vi "FPGAmain_5782_Dual_PID_3.vi"() -> ()   [LabVIEW 2013]
uses:
  FPGA/DataMode.ctl
  FPGA/Input_5782/5782_states.ctl
  <vilib>/Platform/TimedLoop/XDataNode/timing_clust.ctl
  <vilib>/Platform/TimedLoop/XDataNode/nitl_modes.ctl
  <vilib>/Platform/TimedLoop/XDataNode/wakeup.ctl
  <vilib>/rvi/Emulation/niFpgaSctlEmulationGetInTimedLoop.vi
  <vilib>/rvi/Emulation/niFpgaEmulationReportErrorSimple.vi
  <vilib>/rvi/Emulation/niFpgaGetClockAttributes.vi
  <vilib>/rvi/eio/common/nirviEmuTemplateMethod_errors.vi
  <vilib>/rvi/Emulation/niFpgaCriticalErrorInLSC.vi
  <vilib>/rvi/DataTransferAndStorage/Register/Emulation/niFpgaRegisterEmulationFpgaImpl.vi
  <instcachedir>/0/niFpgaRegisterEmulationFpgaImpl_DCF4BC0110594B98B44A971D60CEEC4D.lvgen/niFpgaRegisterEmulationFpgaImpl_DCF4BC0110594B98B44A971D60CEEC4D_005.vi
  <vilib>/rvi/DataTransferAndStorage/Container/Common/niFpgaContainerGetUniqueNameForEmu.vi
  <instcachedir>/0/niFpgaRegisterEmulationFpgaImpl_DCF4BC0110594B98B44A971D60CEEC4D.lvgen/niFpgaRegisterEmulationFpgaImpl_DCF4BC0110594B98B44A971D60CEEC4D_014.vi
  <instcachedir>/0/niFpgaRegisterEmulationFpgaImpl_DCF4BC0110594B98B44A971D60CEEC4D.lvgen/niFpgaRegisterEmulationFpgaImpl_DCF4BC0110594B98B44A971D60CEEC4D_013.vi
  <instcachedir>/0/niFpgaRegisterEmulationFpgaImpl_DCF4BC0110594B98B44A971D60CEEC4D.lvgen/niFpgaRegisterEmulationFpgaImpl_DCF4BC0110594B98B44A971D60CEEC4D_016.vi
  <instcachedir>/0/niFpgaRegisterEmulationFpgaImpl_DCF4BC0110594B98B44A971D60CEEC4D.lvgen/niFpgaRegisterEmulationFpgaImpl_DCF4BC0110594B98B44A971D60CEEC4D_017.vi
  <instcachedir>/0/niFpgaRegisterEmulationFpgaImpl_DCF4BC0110594B98B44A971D60CEEC4D.lvgen/niFpgaRegisterEmulationFpgaImpl_DCF4BC0110594B98B44A971D60CEEC4D_015.vi
  <vilib>/rvi/FIFO/Fifo_Resource/nirvififoEmulationReadFpgaImpl.vi
  <vilib>/rvi/interface/RandomDataEmulation/nirviRandomDataMultiElementFPGAFIFO.vi
  <instcachedir>/0/nirviRandomDataMultiElementFPGAFIFO_F2B80EDE0D7944A08478D8D26097D4DB.lvgen/nirviRandomDataMultiElementFPGAFIFO_F2B80EDE0D7944A08478D8D26097D4DB_005.vi
  <vilib>/rvi/interface/RandomDataEmulation/niFpgaRandomDataHandleErrors.vi
  <instcachedir>/0/niFpgaRegisterEmulationFpgaImpl_DCF4BC0110594B98B44A971D60CEEC4D.lvgen/niFpgaRegisterEmulationFpgaImpl_DCF4BC0110594B98B44A971D60CEEC4D_009.vi
  <vilib>/rvi/interface/RandomDataEmulation/nirviRandomDataFPGAFIFO.vi
  <vilib>/rvi/FIFO/Fifo_Resource/nirvififoEmulationWriteFpgaImpl.vi
  <vilib>/Platform/TimedLoop/XDataNode/XDataNode.xnode
  <vilib>/eio/EIONode/EIONode.xnode
  <vilib>/rvi/DataTransferAndStorage/Container/XNode/niFpgaContainer.xnode
  <vilib>/rvi/DataTransferAndStorage/Register/Emulation/niFpgaRegisterEmulation.vi
  <vilib>/rvi/FIFO/Fifo_Resource/nirvififoEmulationRead.vi
  <vilib>/rvi/interface/RandomDataEmulation/nirviRandomDataFpgaMultiElementTemplate.vi
  <vilib>/rvi/interface/RandomDataEmulation/nirviRandomDataFpgaReadWriteTemplate.vi
  <vilib>/rvi/FIFO/Fifo_Resource/nirvififoEmulationWrite.vi
  <vilib>/Platform/TimedLoop/XDataNode/XDNodeRunTimeDep.lvlib
panel:
  in  "IO Module\\AO Data Sync":bool=TRUE
  in  "IO Module\\SPI Write Data":u16
  out "IO Module\\SPI Read Data":u8
  in  "IO Module\\SPI Read":bool
  in  "IO Module\\SPI Write":bool
  in  "IO Module\\SPI Address":u16
  in  "IO Module\\SPI Device":u8
  out "IO Module\\SPI Idle":bool
  in  "AM phase":fxp<+,64,64>
  in  "delay phase":fxp<+,64,64>
  in  "User Command Commit":bool
  in  "User Command":u8
  out "User Command Idle":bool
  out "User Command Status":u8
  in  "User Data 0":u8
  in  "User Data 1":u8
  out "PLL Locked":bool
  out "User Error":bool
  out "Configured?":bool
  in  "Continuous":bool
  in  "5782 record length":u16=4000 caption="Samples Per Trigger" min=1 step=1
  in  "Trigger Acquisition":bool
  out "IO Module\\Trigger Input":bool
  in  "Downsample":fxp<+,8,8>=1.0
  in  "new coeffs":bool
  in  "FIR coeffs":fxp<+/-,18,18>[](array[numeric])
  in  "CIC Gain":fxp<+/-,32,1>=0.00390625 format="%#_32g"
  in  "Acquisition running":bool
  in  "Phase output":fxp<+,64,64>[](array[numeric])=[0.0, 0.0, 0.0, 0.0, 0.0, 0.0, 0.0, 0.0]
  in  "Simulated phase 5782":fxp<+,64,64>[](array[numeric])=[0.0, 0.0]
  in  "Mode":T1
  in  "Phase 5782":fxp<+,64,64>[](array[numeric])=[0.0, 0.0]
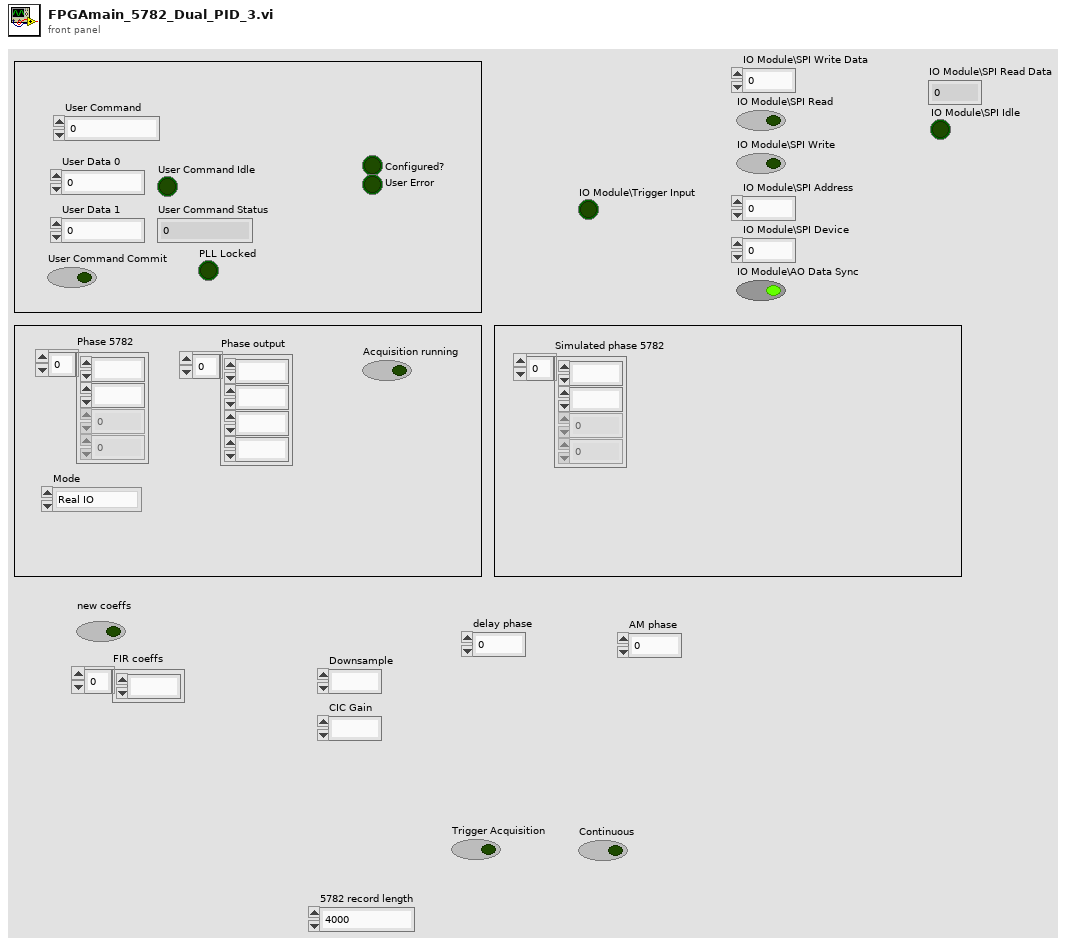
[diagram p1: front panel]
types:
  T1 = typedef "DataMode.ctl" = enum16{"Real IO", "Simulated"}
  T2 = typedef "5782_states.ctl" = enum8{"Wait for trigger", "Acquisition", "Send record length", "Quiet period"}
  T3 = typedef "XDNodeRunTimeDep.lvlib/timing_clust.ctl" = cluster{"Expected End [f-1]":u64, "Actual End [f-1]":u64, "Finished Late? [f-1]":bool, "Expected End [i-1]":u64, "Actual End [i-1]":u64, "Finished Late? [i-1]":bool, "Expected Start [i]":u64, "Actual Start [i]":u64, "Expected Start [f]":u64, "Actual Start [f]":u64, "Source Name":string, "Structure Name":string, "Period":i64, "Deadline":i64, "Offset":i64, "Start":i64, "Priority":i32, "Timeout":i32, "Mode":T4, "Wakeup Reason":T5, "Error":errorcluster, "Source Type":string, "Secondary Source Type":string, "Global End Time":u64, "Global Start Time":u64, "Frame Duration":u64, "Iteration Duration":u64, "Assigned CPU":i32, "I/O Scan Engine Mode":u32}
  T4 = typedef "XDNodeRunTimeDep.lvlib/nitl_modes.ctl" = enum32{"No Change", "Process missed periods, maintain original phase", "Discard missed periods, maintain original phase", "Process missed periods, ignore original phase", "Discard missed periods, ignore original phase"}
  T5 = typedef "XDNodeRunTimeDep.lvlib/wakeup.ctl" = enum32{"Normal", "Aborted", "Asynchronous wakeup", "Timing source error", "Timed loop error", "Timeout"}
  T6 = typedef "I16 array size 2.ctl" = i16[]
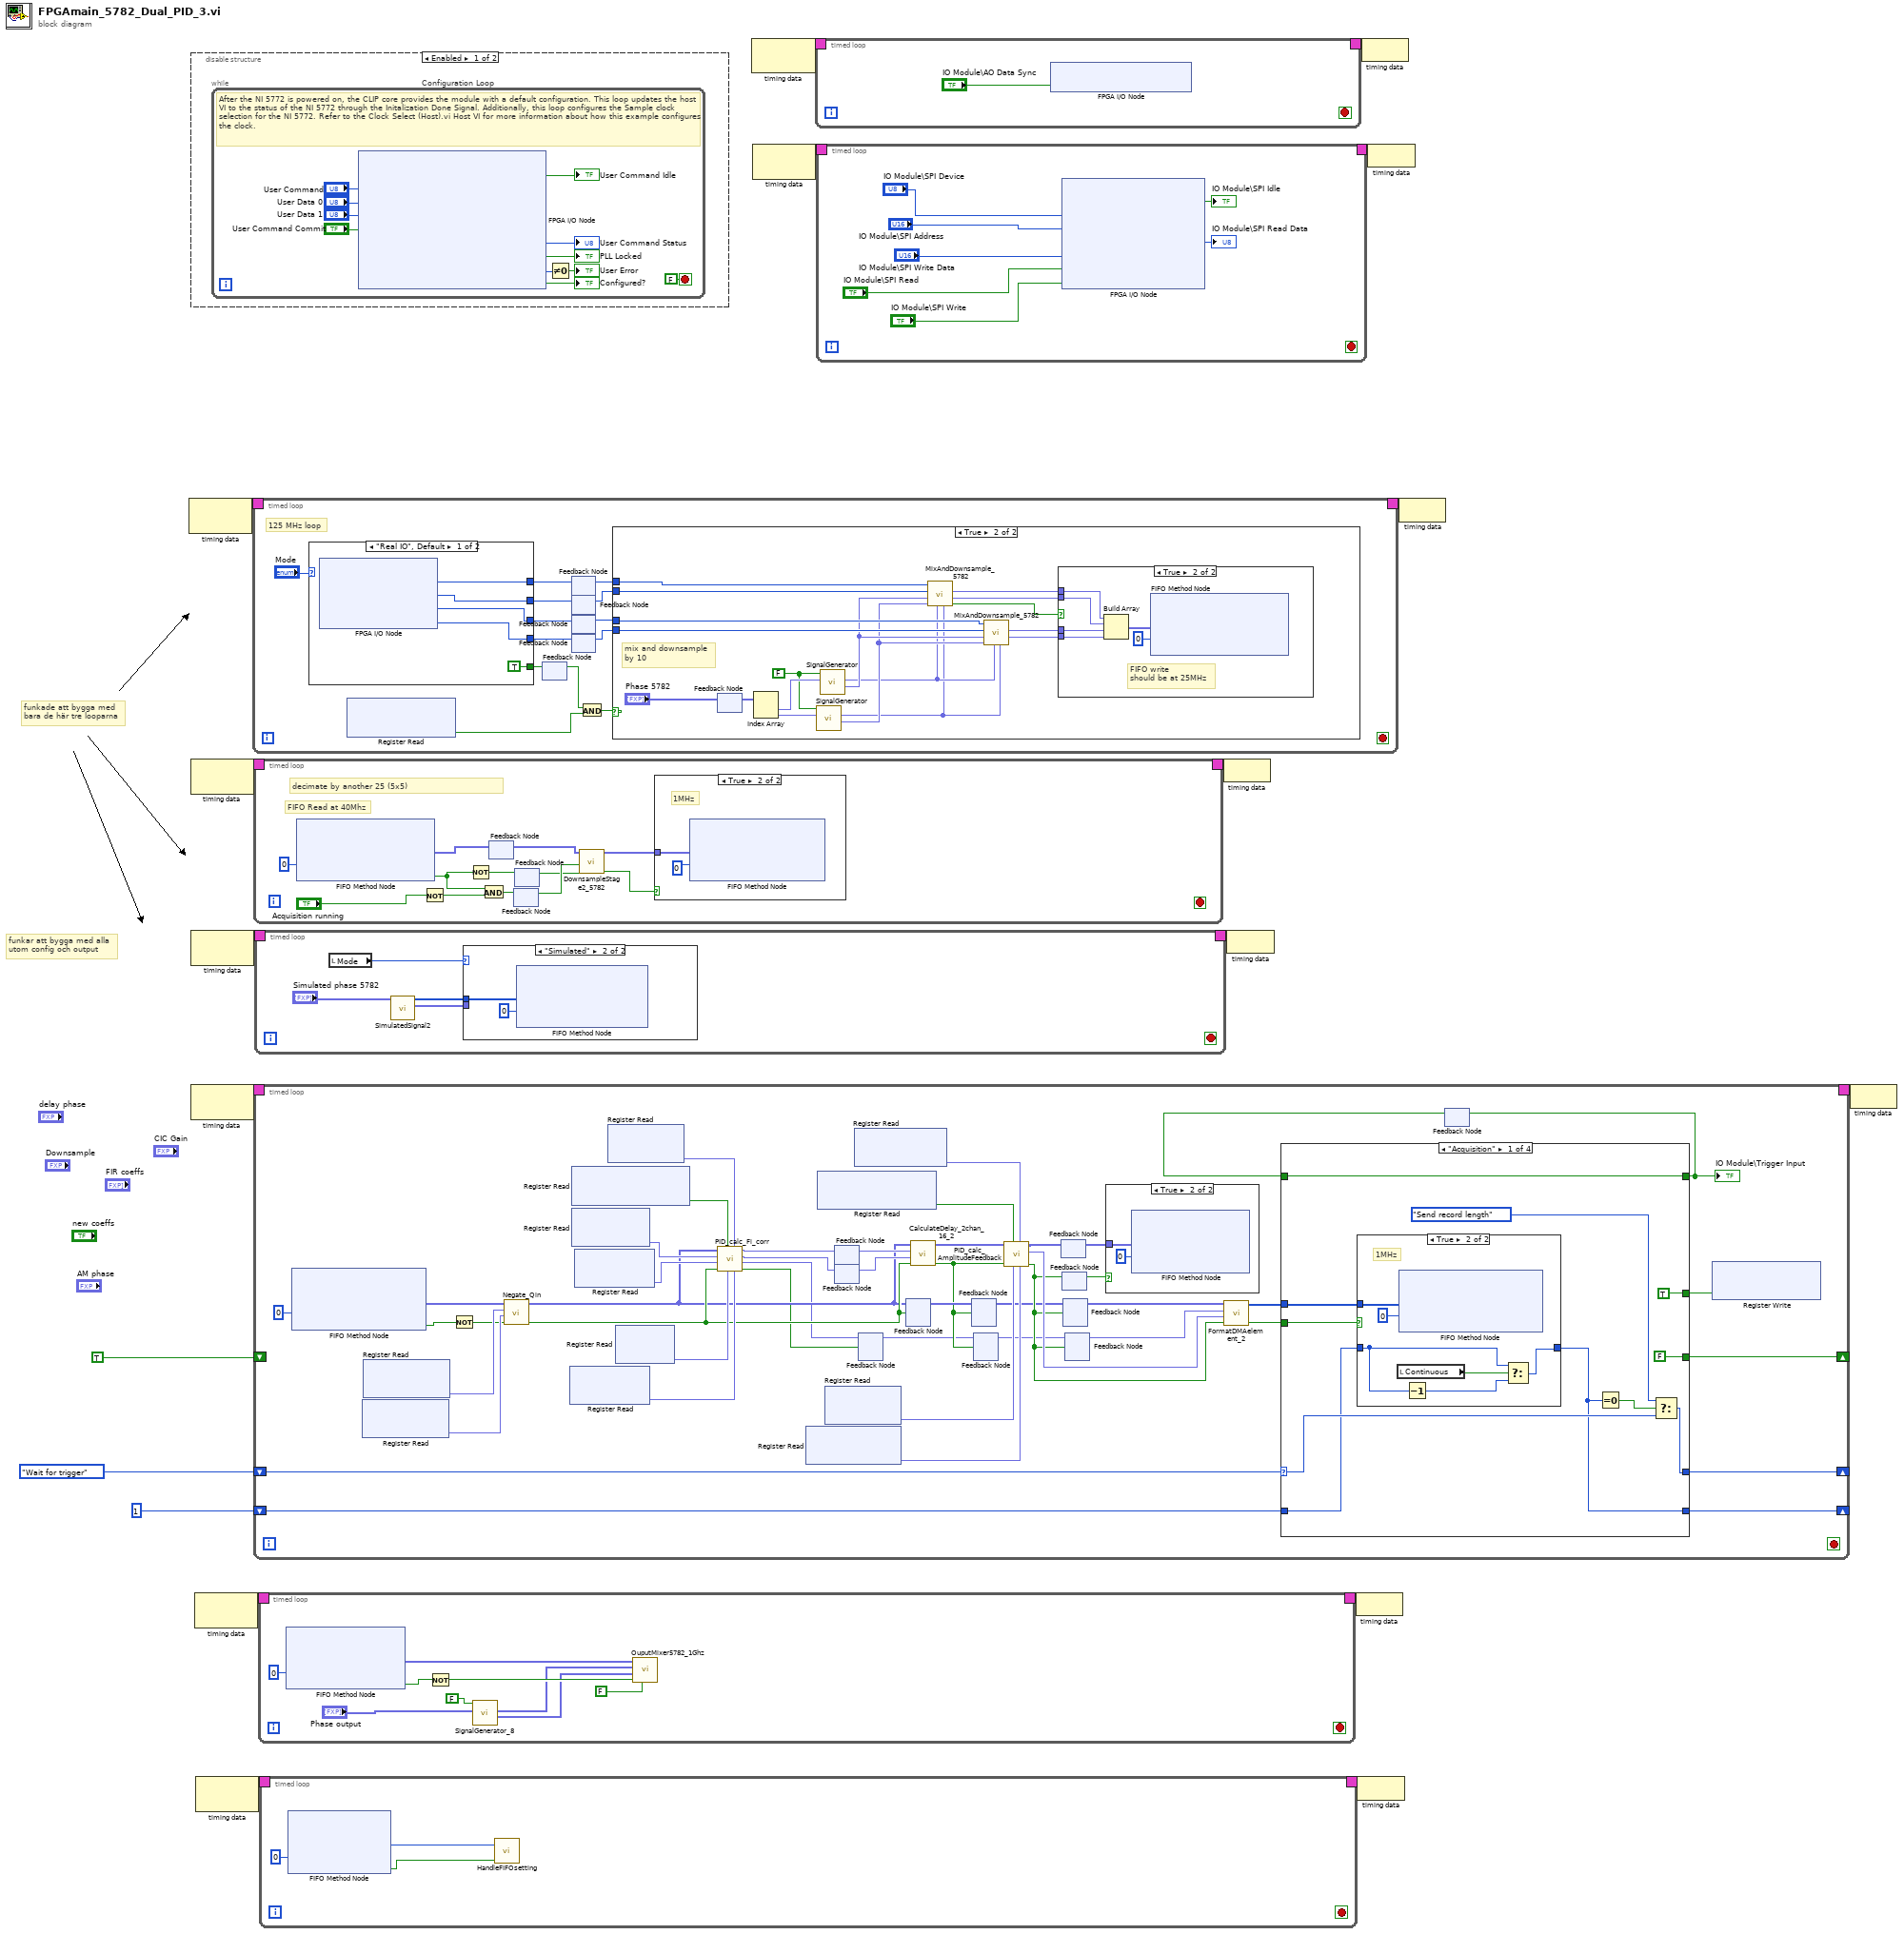
[diagram p0: block diagram]
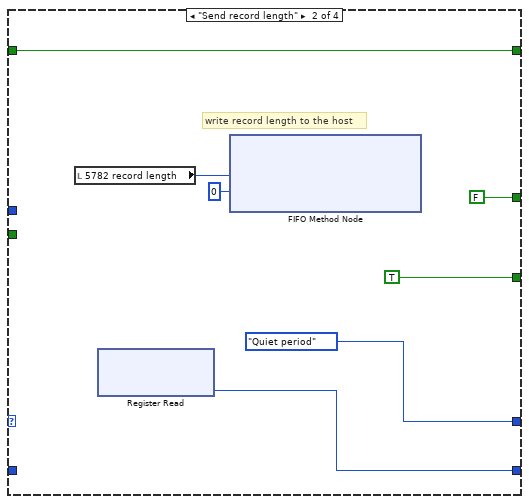
[diagram p4: hidden frame]
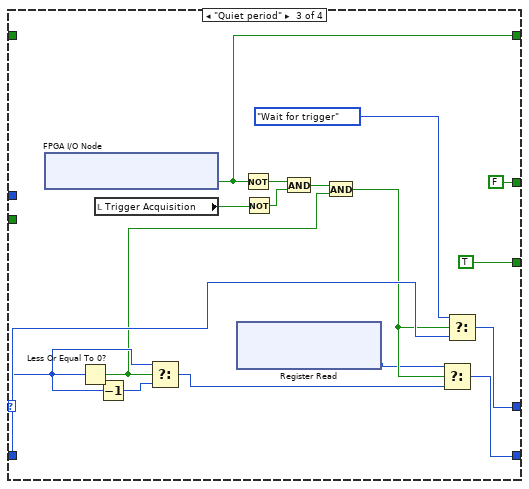
[diagram p5: hidden frame]
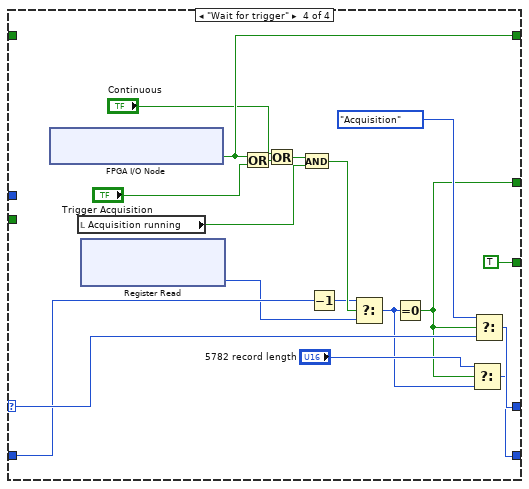
[diagram p6: hidden frame]
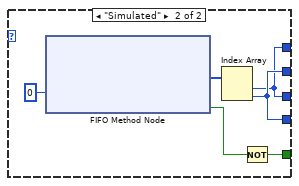
[diagram p10: hidden frame]
diagram:
  # "funkar att bygga med alla\nutom config och output"
  # "funkade att bygga med\nbara de här tre looparna"
  n1 = node-c288() -> (w15:T3)  [unwired: 1 in]
  n2 = disable-structure shown="Enabled" {
    frame Enabled {
      n3 = while "Configuration Loop" {
        stop <- FALSE stop-if-true
        # "After the NI 5772 is powered on, the CLIP core provides the module with a default configuration. This loop updates the host VI to the status of the NI 5772 through the Initalization Done Signal. Additionally, this loop configures the Sample clock selection for the NI 5772. Refer to the Clock Select (Host).vi Host VI for more information about how this example configures the clock."
        n4 = xnode "FPGA I/O Node"("IO Module\\User Command"="User Command", "IO Module\\User Data 0"="User Data 0", "IO Module\\User Data 1"="User Data 1", "IO Module\\User Command Commit"="User Command Commit") -> ("IO Module\\User Command Idle"=→"User Command Idle":bool, "IO Module\\User Command Status"=→"User Command Status":u8, "IO Module\\PLL Locked"=→"PLL Locked":bool, "IO Module\\User Error"=w25:u8, "IO Module\\Initialization Done"=→"Configured?":bool)  [unwired: 9 in, 9 out]
        n5 = Not Equal To 0?(x=w25) -> (x != 0?=→"User Error":bool)
      }
    }
    frame Disabled {
    }
  }
  n6 = node-c288() -> (w19:T3)  [unwired: 1 in]
  n7 = node-c288() -> (w13:T3)  [unwired: 1 in]
  n8 = node-c288() -> (w17:T3)  [unwired: 1 in]
  n9 = node-c288() -> (w6:T3)  [unwired: 1 in]
  n10 = node-c288() -> (w8:T3)  [unwired: 1 in]
  n11 = timed-loop {
    timing: w15 -> [_]
    timing-out: [_] -> w14
    stop <- _ stop-if-true
    # "125 MHz loop"
    n12 = case shown="\"Real IO\", Default" "Mode" {
      tunnel: [w72 w75] -> w41
      tunnel: [w71 w76] -> w39
      tunnel: [w70 w75] -> w37
      tunnel: [w69 w76] -> w34
      tunnel: [TRUE w73] -> w33
      frame "Real IO", Default {
        n13 = xnode "FPGA I/O Node"() -> ("IO Module\\AI 0 N-1"=w72:i16, "IO Module\\AI 0 N"=w71:i16, "IO Module\\AI 1 N-1"=w70:i16, "IO Module\\AI 1 N"=w69:i16)  [unwired: 4 in, 4 out]
      }
      frame "Simulated" {
        n14 = xnode ("FIFO Method Node")("Timeout"=0) -> ("Element"=w77:i16[], "Timed Out?"=w74:bool)  [unwired: 1 in, 1 out]
        n15 = Index Array(array=w77) -> (element #1=w75:i16, element #2=w76:i16)  [unwired: 2 in]
        n16 = Not(x=w74) -> (.not. x?=w73:bool)
      }
    }
    n17 = xnode ("Register Read")() -> ("Data"=w31:bool)  [unwired: 1 in, 1 out]
    n18 = feedback #1() -> (w32:bool)  [unwired: 1 in]
    n19 = feedback-in #1(w33) -> ()
    n20 = feedback #2() -> (w40:i16)  [unwired: 1 in]
    n21 = feedback-in #2(w41) -> ()
    n22 = feedback #3() -> (w38:i16)  [unwired: 1 in]
    n23 = feedback-in #3(w39) -> ()
    n24 = feedback #4() -> (w36:i16)  [unwired: 1 in]
    n25 = feedback-in #4(w37) -> ()
    n26 = feedback #5() -> (w35:i16)  [unwired: 1 in]
    n27 = feedback-in #5(w34) -> ()
    n28 = And(x=w32, y=w31) -> (x .and. y?=w42:bool)
    n29 = case shown="True" w42 {
      tunnel: w40 -> [_ w51]
      tunnel: w38 -> [_ w50]
      tunnel: w36 -> [_ w49]
      tunnel: w35 -> [_ w48]
      frame False {
      }
      frame True {
        w52 = FALSE
        # "mix and downsample\nby 10"
        n30 = feedback #6() -> (w55:fxp<+,64,64>[])  [unwired: 1 in]
        n31 = feedback-in #6("Phase 5782") -> ()
        n32 = Index Array(array=w55) -> (element #1=w54:fxp<+,64,64>, element #2=w56:fxp<+,64,64>)  [unwired: 2 in]
        n33 = call "SignalGenerator.vi"("phase"=w56, "Reset"=w52) -> ("Cos"=w46:fxp<+/-,16,0>, "Sin"=w44:fxp<+/-,16,0>)  [unwired: 7 in, 1 out]
        n34 = call "SignalGenerator.vi"("phase"=w54, "Reset"=w52) -> ("Cos"=w47:fxp<+/-,16,0>, "Sin"=w45:fxp<+/-,16,0>)  [unwired: 7 in, 1 out]
        n35 = call "MixAndDownsample_5782.vi"("sin1"=w44, "sin0"=w45, "cos1"=w46, "cos0"=w47, "signal 1"=w50, "signal 0"=w51) -> ("data valid"=w59:bool, "Q out"=w60:fxp<+/-,16,14>, "I out"=w61:fxp<+/-,16,14>)  [unwired: 3 in]
        n36 = call "MixAndDownsample_5782.vi"("sin1"=w44, "sin0"=w45, "cos1"=w46, "cos0"=w47, "signal 1"=w48, "signal 0"=w49) -> ("Q out"=w57:fxp<+/-,16,14>, "I out"=w58:fxp<+/-,16,14>)  [unwired: 3 in, 1 out]
        n37 = case shown="True" w59 {
          tunnel: w60 -> [_ w67]
          tunnel: w61 -> [_ w64]
          tunnel: w58 -> [_ w63]
          tunnel: w57 -> [_ w62]
          frame False {
          }
          frame True {
            # "FIFO write\nshould be at 25MHz"
            n38 = Build Array(w64, w67, w63, w62) -> (w66:fxp<+/-,16,14>[])
            n39 = xnode ("FIFO Method Node")("Element"=w66, "Timeout"=0) -> ()  [unwired: 1 in, 2 out]
          }
        }
      }
    }
  }
  n40 = timed-loop {
    timing: w19 -> [_]
    timing-out: [_] -> w18
    stop <- _ stop-if-true
    # "FIFO Read at 40Mhz"
    # "decimate by another 25 (5x5)"
    n41 = xnode ("FIFO Method Node")("Timeout"=0) -> ("Element"=w86:fxp<+/-,16,14>[], "Timed Out?"=w88:bool)  [unwired: 1 in, 1 out]
    n42 = Not(x="Acquisition running") -> (.not. x?=w89:bool)
    n43 = Not(x=w88) -> (.not. x?=w82:bool)
    n44 = And(x=w88, y=w89) -> (x .and. y?=w84:bool)
    n45 = feedback #7() -> (w85:fxp<+/-,16,14>[])  [unwired: 1 in]
    n46 = feedback-in #7(w86) -> ()
    n47 = feedback #8() -> (w83:bool)  [unwired: 1 in]
    n48 = feedback-in #8(w84) -> ()
    n49 = feedback #9() -> (w81:bool)  [unwired: 1 in]
    n50 = feedback-in #9(w82) -> ()
    n51 = call "DownsampleStage2_5782.vi"("valid in"=w81, "reset"=w83, "Data in"=w85) -> ("valid out"=w90:bool, "data out"=w91:fxp<+/-,16,14>[])  [unwired: 7 in]
    n52 = case shown="True" w90 {
      tunnel: w91 -> [_ w93]
      frame False {
      }
      frame True {
        # "1MHz"
        n53 = xnode ("FIFO Method Node")("Element"=w93, "Timeout"=0) -> ()  [unwired: 1 in, 2 out]
      }
    }
  }
  n54 = timed-loop {
    timing: w13 -> [_]
    timing-out: [_] -> w12
    shift-right: [w141] -> _
    shift-left: 5782_states."Wait for trigger" ("5782 states") -> [w143]
    shift-right: [w140] -> _
    shift-left: u16 1 ("trigger samples") -> [w142]
    shift-right: [w135] -> _
    shift-left: TRUE -> [_]
    stop <- _ stop-if-true
    n55 = xnode ("FIFO Method Node")("Timeout"=0) -> ("Element"=w121:fxp<+/-,16,14>[], "Timed Out?"=w138:bool)  [unwired: 1 in, 1 out]
    n56 = xnode ("Register Read")() -> ("Data"=w128:fxp<+/-,16,14>)  [unwired: 1 in, 1 out]
    n57 = xnode ("Register Read")() -> ("Data"=w129:fxp<+/-,16,14>)  [unwired: 1 in, 1 out]
    n58 = Not(x=w138) -> (.not. x?=w122:bool)
    n59 = call "Negate_Qin.vi"("valid in"=w122, "DC offset chan 1"=w128, "DC offset chan 0"=w129, "Data in"=w121) -> ("valid out"=w107:bool, "Data out"=w106:fxp<+/-,16,14>[])  [unwired: 6 in]
    n60 = xnode "Register Read"() -> ("Data"=w114:fxp<+/-,32,4>)  [unwired: 1 in, 1 out]
    n61 = xnode "Register Read"() -> ("Data"=w111:bool)  [unwired: 1 in, 1 out]
    n62 = xnode "Register Read"() -> ("Data"=w112:fxp<+/-,32,4>)  [unwired: 1 in, 1 out]
    n63 = xnode "Register Read"() -> ("Data"=w113:fxp<+/-,32,4>)  [unwired: 1 in, 1 out]
    n64 = xnode "Register Read"() -> ("Data"=w110:fxp<+/-,32,4>)  [unwired: 1 in, 1 out]
    n65 = xnode "Register Read"() -> ("Data"=w115:fxp<+/-,32,4>)  [unwired: 1 in, 1 out]
    n66 = call "PID_calc_Fi_corr.vi"("Kd/Tau"=w114, "Ki*Tau"=w110, "Kp"=w115, "Enabled"=w111, "input valid"=w107, "Fi_delta"=w113, "Fi_start"=w112, "Data in"=w106) -> ("output valid"=w104:bool, "c out"=w105:fxp<+/-,32,4>, "cos_fi_korr"=w108:fxp<+/-,16,2>, "sin fi_korr"=w109:fxp<+/-,16,2>)
    n67 = xnode ("Register Read")() -> ("Data"=w124:fxp<+/-,32,6>)  [unwired: 1 in, 1 out]
    n68 = xnode ("Register Read")() -> ("Data"=w126:bool)  [unwired: 1 in, 1 out]
    n69 = xnode ("Register Read")() -> ("Data"=w125:fxp<+/-,32,6>)  [unwired: 1 in, 1 out]
    n70 = feedback-in #10(w109) -> ()
    n71 = feedback #10() -> (w131:fxp<+/-,16,2>)  [unwired: 1 in]
    n72 = feedback #11() -> (w130:fxp<+/-,16,2>)  [unwired: 1 in]
    n73 = feedback-in #11(w108) -> ()
    n74 = xnode ("Register Read")() -> ("Data"=w123:fxp<+/-,32,6>)  [unwired: 1 in, 1 out]
    n75 = feedback #12() -> (w98:fxp<+/-,32,4>)  [unwired: 1 in]
    n76 = feedback-in #12(w105, w104) -> ()
    n77 = feedback #13() -> (w101:fxp<+/-,16,14>[])  [unwired: 1 in]
    n78 = feedback-in #13(w106, w107) -> ()
    n79 = call "CalculateDelay_2chan_16_2.vi"("input valid"=w107, "cos_fi"=w130, "sin fi"=w131, "Data in"=w106) -> ("output valid"=w99:bool, "Data out"=w127:fxp<+/-,16,14>[])  [unwired: 6 in]
    n80 = feedback #14() -> (w100:fxp<+/-,16,14>[])  [unwired: 1 in]
    n81 = feedback-in #14(w101, w99) -> ()
    n82 = feedback #15() -> (w97:fxp<+/-,32,4>)  [unwired: 1 in]
    n83 = feedback-in #15(w98, w99) -> ()
    n84 = call "PID_calc_AmplitudeFeedback.vi"("Kd/Tau"=w124, "Ki*Tau"=w123, "Kp"=w125, "Enabled"=w126, "input valid"=w99, "Data in"=w127) -> ("output valid"=w103:bool, "c(t)"=w116:fxp<+/-,32,21>, "data out"=w120:fxp<+/-,16,14>[])  [unwired: 2 in, 1 out]
    n85 = feedback #16() -> (w119:fxp<+/-,16,14>[])  [unwired: 1 in]
    n86 = feedback-in #16(w120) -> ()
    n87 = feedback #17() -> (w118:bool)  [unwired: 1 in]
    n88 = feedback-in #17(w103) -> ()
    n89 = feedback #18() -> (w117:fxp<+/-,16,14>[])  [unwired: 1 in]
    n90 = feedback-in #18(w100, w103) -> ()
    n91 = feedback #19() -> (w102:fxp<+/-,32,4>)  [unwired: 1 in]
    n92 = feedback-in #19(w97, w103) -> ()
    n93 = case shown="True" w118 {
      tunnel: w119 -> [_ w144]
      frame False {
      }
      frame True {
        n94 = xnode ("FIFO Method Node")("Element"=w144, "Timeout"=0) -> ()  [unwired: 1 in, 2 out]
      }
    }
    n95 = call "FormatDMAelement_2.vi"("valid in"=w103, "c(t) - AM"=w116, "c(t) - Phase"=w102, "Data in"=w117) -> ("valid out"=w136:bool, "Element"=w137:u64[])  [unwired: 6 in]
    n96 = feedback #20() -> (w133:bool)  [unwired: 1 in]
    n97 = case shown="\"Acquisition\"" w143 {
      selector: w143 -> [w156 _ w186 w205]
      tunnel: w142 -> [w152 _ w174 w192]
      tunnel: [w155 5782_states."Quiet period" ("5782 states") w185 w204] -> w141
      tunnel: [w149 w164 w187 w203] -> w140
      tunnel: w137 -> [w150 _ _ _]
      tunnel: w136 -> [w151 _ _ _]
      tunnel: [FALSE TRUE TRUE TRUE] -> w135
      tunnel: [TRUE FALSE ("5782 triggered") FALSE ("5782 triggered") w196] -> w134
      tunnel: [w148 w165 w176 w195] -> w132
      tunnel: w133 -> [w148 w165 _ _]
      frame "Acquisition" {
        n98 = case shown="True" w151 {
          tunnel: w150 -> [_ w163]
          tunnel: [w157 w160] -> w149
          tunnel: w152 -> [w157 w158]
          frame False {
          }
          frame True {
            # "1MHz"
            n99 = local read "Continuous"() -> (w161:bool)
            n100 = xnode ("FIFO Method Node")("Element"=w163, "Timeout"=0) -> ()  [unwired: 1 in, 2 out]
            n101 = Decrement(x=w158) -> (x-1=w159:u16)
            n102 = Select(t=w158, s=w161, f=w159) -> (s? t:f=w160:u16)
          }
        }
        n103 = Equal To 0?(x=w149) -> (x = 0?=w153:bool)
        n104 = Select(t=5782_states."Send record length" ("5782 states"), s=w153, f=w156) -> (s? t:f=w155:T2)
      }
      frame "Send record length" {
        # "write record length to the host"
        n105 = local read "5782 record length"() -> (w167:u16)
        n106 = xnode ("Register Read")() -> ("Data"=w164:u16)  [unwired: 1 in, 1 out]
        n107 = xnode ("FIFO Method Node")("Element"=w167, "Timeout"=0) -> ()  [unwired: 1 in, 2 out]
      }
      frame "Quiet period" {
        n108 = xnode "FPGA I/O Node"() -> ("IO Module\\Trigger Input"=w176:bool)  [unwired: 1 in, 1 out]
        n109 = Less Or Equal To 0?(x=w174) -> (x <= 0?=w173:bool)
        n110 = local read "Trigger Acquisition"() -> (w182:bool)
        n111 = Decrement(x=w174) -> (x-1=w175:u16)
        n112 = Select(t=w174, s=w173, f=w175) -> (s? t:f=w172:u16)
        n113 = xnode ("Register Read")() -> ("Data"=w171:u16)  [unwired: 1 in, 1 out]
        n114 = Not(x=w176) -> (.not. x?=w181:bool)
        n115 = Not(x=w182) -> (.not. x?=w180:bool)
        n116 = And(x=w181, y=w180) -> (x .and. y?=w179:bool)
        n117 = And(x=w179, y=w173) -> (x .and. y?=w184:bool)
        n118 = Select(t=w171, s=w184, f=w172) -> (s? t:f=w187:u16)
        n119 = Select(t=5782_states."Wait for trigger" ("5782 states"), s=w184, f=w186) -> (s? t:f=w185:T2)
      }
      frame "Wait for trigger" {
        n120 = xnode "FPGA I/O Node"() -> ("IO Module\\Trigger Input"=w195:bool)  [unwired: 1 in, 1 out]
        n121 = local read "Acquisition running"() -> (w197:bool)
        n122 = xnode ("Register Read")() -> ("Data"=w188:u16)  [unwired: 1 in, 1 out]
        n123 = Or(x=w195, y="Trigger Acquisition") -> (x .or. y?=w191:bool)
        n124 = Or(x="Continuous", y=w191) -> (x .or. y?=w189:bool)
        n125 = And(x=w189, y=w197) -> (x .and. y?=w198:bool)
        n126 = Decrement(x=w192) -> (x-1=w193:u16)
        n127 = Select(t=w193, s=w198, f=w188) -> (s? t:f=w194:u16)
        n128 = Equal To 0?(x=w194) -> (x = 0?=w196:bool)
        n129 = Select(t="5782 record length", s=w196, f=w194) -> (s? t:f=w203:u16)
        n130 = Select(t=5782_states."Acquisition" ("5782 states"), s=w196, f=w205) -> (s? t:f=w204:T2)
      }
    }
    "IO Module\\Trigger Input" <- w132
    n131 = feedback-in #20(w132) -> ()
    n132 = xnode ("Register Write")("Data"=w134) -> ()  [unwired: 1 in, 1 out]
  }
  n133 = timed-loop {
    timing: w17 -> [_]
    timing-out: [_] -> w16
    stop <- _ stop-if-true
    n134 = local read "Mode"() -> (w211:T1)
    n135 = call "SimulatedSignal2.vi"("Phase"="Simulated phase 5782") -> ("dummy do not use"=w208:fxp<+/-,16,0>[], "output"=w210:T6)  [unwired: 9 in]
    n136 = case shown="\"Simulated\"" w211 {
      tunnel: w210 -> [_ w212]
      tunnel: w208 -> [_ _]
      frame "Real IO", Default {
      }
      frame "Simulated" {
        n137 = xnode ("FIFO Method Node")("Element"=w212, "Timeout"=0) -> ()  [unwired: 1 in, 2 out]
      }
    }
  }
  n138 = timed-loop {
    timing: w6 -> [_]
    timing-out: [_] -> w5
    stop <- _ stop-if-true
    n139 = xnode ("FIFO Method Node")("Timeout"=0) -> ("Element"=w220:fxp<+/-,16,14>[], "Timed Out?"=w223:bool)  [unwired: 1 in, 1 out]
    n140 = Not(x=w223) -> (.not. x?=w219:bool)
    n141 = call "SignalGenerator_8.vi"("Phase"="Phase output", "reset"=FALSE) -> ("Sine out"=w216:fxp<+/-,16,0>[], "Cosine out"=w217:fxp<+/-,16,0>[])  [unwired: 8 in]
    n142 = call "OuputMixer5782_1Ghz.vi"("reset"=FALSE, "valid in"=w219, "Sine in"=w216, "Cosine in"=w217, "Data in"=w220) -> ()  [unwired: 5 in, 2 out]
  }
  n143 = timed-loop {
    timing: w8 -> [_]
    timing-out: [_] -> w7
    stop <- _ stop-if-true
    n144 = xnode ("FIFO Method Node")("Timeout"=0) -> ("Element"=w228:u64, "Timed Out?"=w227:bool)  [unwired: 1 in, 1 out]
    n145 = call "HandleFIFOsetting.vi"("timed out"=w227, "Value"=w228) -> ()  [unwired: 10 in]
  }
  n146 = node-c288() -> (w2:T3)  [unwired: 1 in]
  n147 = node-c288() -> (w4:T3)  [unwired: 1 in]
  n148 = timed-loop {
    timing: w2 -> [_]
    timing-out: [_] -> w1
    stop <- _ stop-if-true
    n149 = xnode "FPGA I/O Node"("IO Module\\AO Data Sync"="IO Module\\AO Data Sync") -> ()  [unwired: 1 in, 1 out]
  }
  n150 = timed-loop {
    timing: w4 -> [_]
    timing-out: [_] -> w3
    stop <- _ stop-if-true
    n151 = xnode "FPGA I/O Node"("IO Module\\SPI Device"="IO Module\\SPI Device", "IO Module\\SPI Address"="IO Module\\SPI Address", "IO Module\\SPI Write Data"="IO Module\\SPI Write Data", "IO Module\\SPI Read"="IO Module\\SPI Read", "IO Module\\SPI Write"="IO Module\\SPI Write") -> ("IO Module\\SPI Idle"=→"IO Module\\SPI Idle":bool, "IO Module\\SPI Read Data"=→"IO Module\\SPI Read Data":u8)  [unwired: 7 in, 7 out]
  }
  n152 = node-c288(w18) -> ()
  n153 = node-c288(w16) -> ()
  n154 = node-c288(w5) -> ()
  n155 = node-c288(w7) -> ()
  n156 = node-c288(w1) -> ()
  n157 = node-c288(w3) -> ()
  n158 = node-c288(w14) -> ()
  n159 = node-c288(w12) -> ()
